vi "GEOM_MergeROIs.vi"(9 "curr rois":T2, 10 "new roi":T3={"xstart"=1, "ystart"=1, "xsize"=1, "ysize"=1}) -> (1 "rois out":T1(array[cluster]))   [LabVIEW 2016]
uses:
  GEOM_Coords.ctl
  GEOM_ROI.ctl
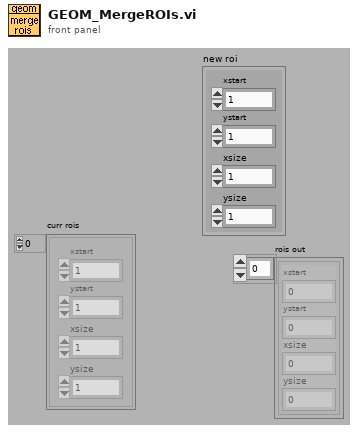
[diagram p1: front panel]
types:
  T1 = cluster{"xstart":i32, "ystart":i32, "xsize":i32, "ysize":i32}[]
  T2 = typedef "GEOM_ROI.ctl" = T3[]
  T3 = typedef "GEOM_Coords.ctl" = cluster{"xstart":u32, "ystart":u32, "xsize":u32, "ysize":u32}
  T4 = cluster{"xstart":i32, "ystart":i32, "xend":i32, "yend":i32}
  T5 = cluster{"xstart":i32, "ystart":i32, "xsize":i32, "ysize":i32}
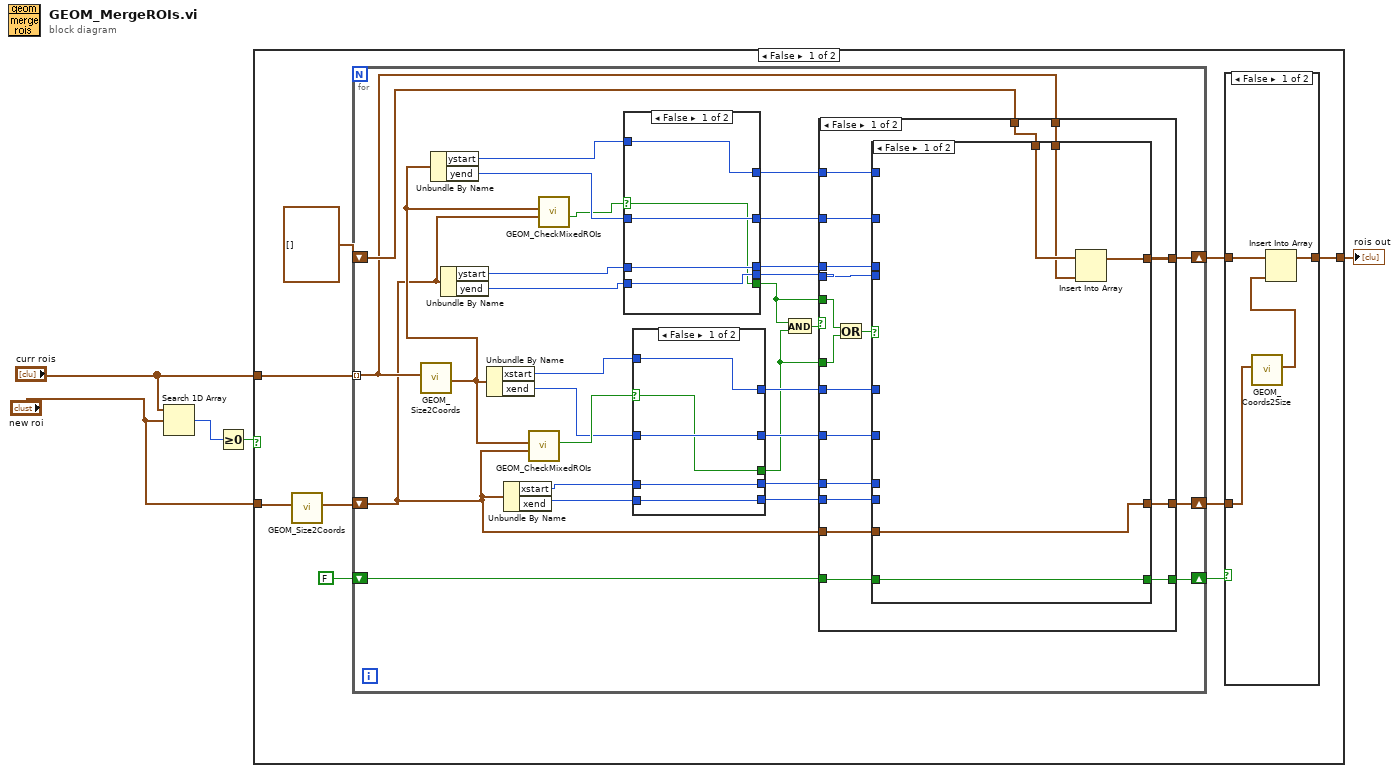
[diagram p0: block diagram]
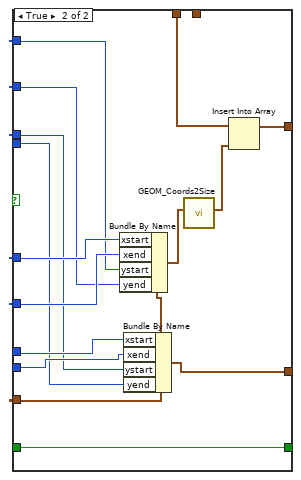
[diagram p3: hidden frame]
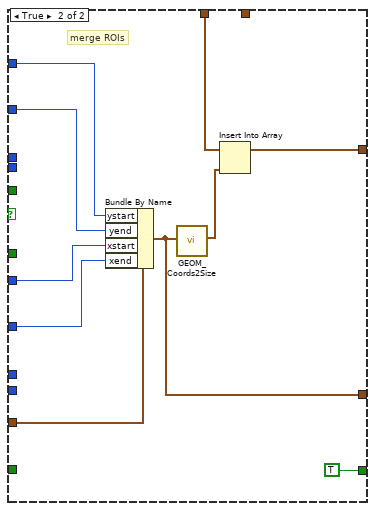
[diagram p4: hidden frame]
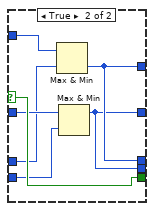
[diagram p5: hidden frame]
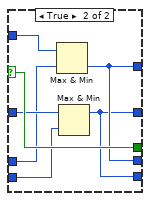
[diagram p6: hidden frame]
diagram:
  n1 = Search 1D Array(1D array="curr rois", element="new roi") -> (index of element=w5:i32)  [unwired: 1 out]
  n2 = Greater Or Equal To 0?(x=w5) -> (x >= 0?=w2:bool)
  n3 = case shown="False" w2 {
    tunnel: "new roi" -> [w8 _]
    tunnel: "curr rois" -> [w14 w121]
    tunnel: [w10 w121] -> w1
    frame False {
      n4 = call "GEOM_Size2Coords.vi"("Size"=w8) -> ("Coords"=w7:T4)  [unwired: 10 out]
      n5 = for {
        tunnel: w14 -> [w33] mode=indexing
        shift-right: [w41] -> w11
        shift-left: T1 [] -> [w40]
        shift-right: [w31] -> w9
        shift-left: w7 -> [w21]
        shift-right: [w32] -> w12
        shift-left: FALSE -> [w20]
        n6 = call "GEOM_Size2Coords.vi"("Size"=w33) -> ("Coords"=w22:T4)  [unwired: 10 out]
        n7 = Unbundle By Name(w22) -> ("ystart"=w25:i32, "yend"=w24:i32)
        n8 = Unbundle By Name(w21) -> ("ystart"=w27:i32, "yend"=w26:i32)
        n9 = Unbundle By Name(w22) -> ("xstart"=w29:i32, "xend"=w28:i32)
        n10 = Unbundle By Name(w21) -> ("xstart"=w48:i32, "xend"=w47:i32)
        n11 = call "GEOM_CheckMixedROIs.vi"("roi coord2"=w21, "roi coord1"=w22) -> ("x mixed"=w30:bool)  [unwired: 9 out]
        n12 = call "GEOM_CheckMixedROIs.vi"("roi coord2"=w21, "roi coord1"=w22) -> ("y mixed"=w23:bool)  [unwired: 9 out]
        n13 = case shown="False" w23 {
          selector: w23 -> [w97 w108]
          tunnel: w27 -> [w99 w105]
          tunnel: w25 -> [w101 w107]
          tunnel: w26 -> [w98 w104]
          tunnel: w24 -> [w100 w106]
          tunnel: [w101 w103] -> w43
          tunnel: [w100 w102] -> w42
          tunnel: [w97 w108] -> w34
          tunnel: [w99 w103] -> w36
          tunnel: [w98 w102] -> w35
          frame False {
          }
          frame True {
            n14 = Max & Min(x=w107, y=w105) -> (min(x,y)=w103:i32)  [unwired: 1 out]
            n15 = Max & Min(x=w106, y=w104) -> (max(x,y)=w102:i32)  [unwired: 1 out]
          }
        }
        n16 = case shown="False" w30 {
          selector: w30 -> [w109 w120]
          tunnel: w48 -> [w111 w117]
          tunnel: w29 -> [w113 w119]
          tunnel: w47 -> [w110 w116]
          tunnel: w28 -> [w112 w118]
          tunnel: [w113 w115] -> w45
          tunnel: [w112 w114] -> w44
          tunnel: [w109 w120] -> w39
          tunnel: [w111 w115] -> w38
          tunnel: [w110 w114] -> w37
          frame False {
          }
          frame True {
            n17 = Max & Min(x=w119, y=w117) -> (min(x,y)=w115:i32)  [unwired: 1 out]
            n18 = Max & Min(x=w118, y=w116) -> (max(x,y)=w114:i32)  [unwired: 1 out]
          }
        }
        n19 = And(x=w34, y=w39) -> (x .and. y?=w46:bool)
        n20 = case shown="False" w46 {
          tunnel: w45 -> [w66 w93]
          tunnel: w44 -> [w65 w92]
          tunnel: w43 -> [w57 w95]
          tunnel: w42 -> [w56 w94]
          tunnel: w21 -> [w62 w96]
          tunnel: [w58 w91] -> w41
          tunnel: w40 -> [w59 w90]
          tunnel: w39 -> [w54 _]
          tunnel: w38 -> [w64 _]
          tunnel: w37 -> [w63 _]
          tunnel: w36 -> [w61 _]
          tunnel: w35 -> [w60 _]
          tunnel: w34 -> [w55 _]
          tunnel: [w52 TRUE] -> w32
          tunnel: w33 -> [w51 _]
          tunnel: [w50 w87] -> w31
          tunnel: w20 -> [w49 _]
          frame False {
            n21 = Or(x=w55, y=w54) -> (x .or. y?=w53:bool)
            n22 = case shown="False" w53 {
              tunnel: w66 -> [_ w86]
              tunnel: w65 -> [_ w85]
              tunnel: w64 -> [_ w84]
              tunnel: w63 -> [_ w83]
              tunnel: w62 -> [w68 w82]
              tunnel: w61 -> [_ w81]
              tunnel: w60 -> [_ w80]
              tunnel: w59 -> [w71 w79]
              tunnel: [w70 w75] -> w58
              tunnel: w57 -> [_ w78]
              tunnel: w56 -> [_ w77]
              tunnel: [w67 w72] -> w52
              tunnel: w51 -> [w69 _]
              tunnel: [w68 w76] -> w50
              tunnel: w49 -> [w67 w72]
              frame False {
                n23 = Insert Into Array(array=w71, new element=w69) -> (w70:T1)  [unwired: 1 in]
              }
              frame True {
                n24 = Bundle By Name(cluster=w82, "xstart"=w86, "xend"=w85, "ystart"=w78, "yend"=w77) -> (w74:T4)
                n25 = Bundle By Name(cluster=w82, "xstart"=w84, "xend"=w83, "ystart"=w81, "yend"=w80) -> (w76:T4)
                n26 = call "GEOM_Coords2Size.vi"("Coords"=w74) -> ("Size"=w73:T5)  [unwired: 10 out]
                n27 = Insert Into Array(array=w79, new element=w73) -> (w75:T1)  [unwired: 1 in]
              }
            }
          }
          frame True {
            # "merge ROIs"
            n28 = Bundle By Name(cluster=w96, "ystart"=w95, "yend"=w94, "xstart"=w93, "xend"=w92) -> (w87:T4)
            n29 = call "GEOM_Coords2Size.vi"("Coords"=w87) -> ("Size"=w88:T5)  [unwired: 10 out]
            n30 = Insert Into Array(array=w90, new element=w88) -> (w91:T1)  [unwired: 1 in]
          }
        }
      }
      n31 = case shown="False" w12 {
        tunnel: w11 -> [w18 w19]
        tunnel: [w17 w19] -> w10
        tunnel: w9 -> [w16 _]
        frame False {
          n32 = call "GEOM_Coords2Size.vi"("Coords"=w16) -> ("Size"=w15:T5)  [unwired: 10 out]
          n33 = Insert Into Array(array=w18, new element=w15) -> (w17:T1)  [unwired: 1 in]
        }
        frame True {
        }
      }
    }
    frame True {
    }
  }
  "rois out" <- w1
